vi "Untitled 1.vi"() -> ()   [LabVIEW 2014]
uses:
  <vilib>/addons/control/pid/NI_PID_pid.lvlib
  <vilib>/addons/control/pid/pid.llb/PID (DBL).vi
panel:
  out "Inches Desired 2":dbl
  in  "stop":bool
  out "In Range? 2":bool
  out "Interpolation Error 2":dbl format="%0.2f"
  out "Seconds for Traversal 2":dbl format="%0.2f"
  in  "Inches Desired":dbl(slide) scale=0.0..100.0
  out "Time Required (sec)":dbl
  in  "Distance to Travel (m)":dbl
  out "In Range?":bool
  out "Interpolation Error":dbl format="%0.2f"
  out "Seconds for Traversal":dbl format="%0.2f"
  in  "Watts Available":dbl=1000.0 format="%0.2f"
  in  "PID gains":T1={"proportional gain (Kc)"=1.0, "integral time (Ti, min)"=0.01, "derivative time (Td, min)"=0.0}
  in  "output range":cluster{"output high":dbl, "output low":dbl}={"output high"=1.0, "output low"=0.0}
  in  "process variable":dbl format="%.2f"
  in  "setpoint":dbl format="%.2f"
  out "output to motor":dbl format="%.2f"
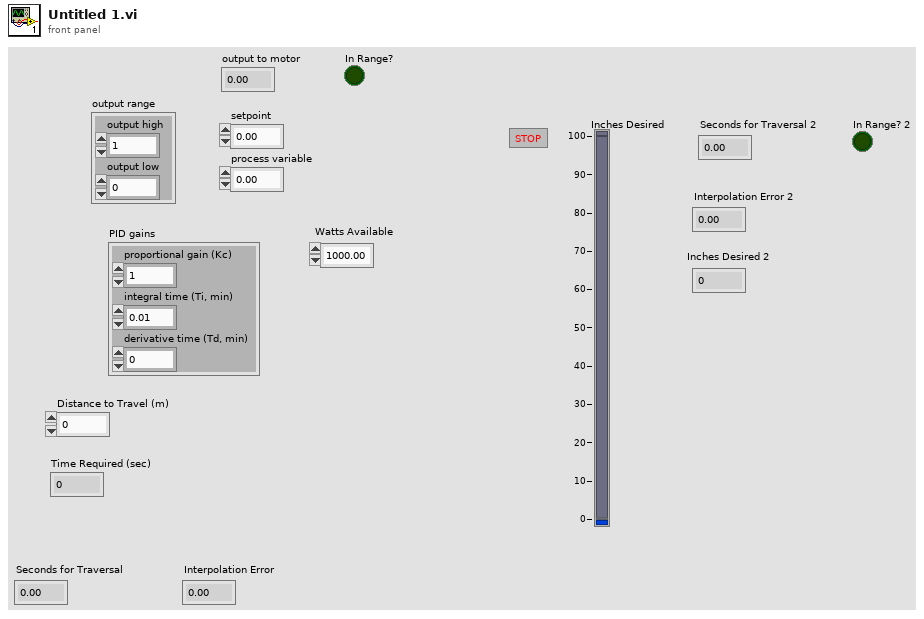
[diagram p1: front panel]
types:
  T1 = cluster{"proportional gain (Kc)":dbl, "integral time (Ti, min)":dbl, "derivative time (Td, min)":dbl}
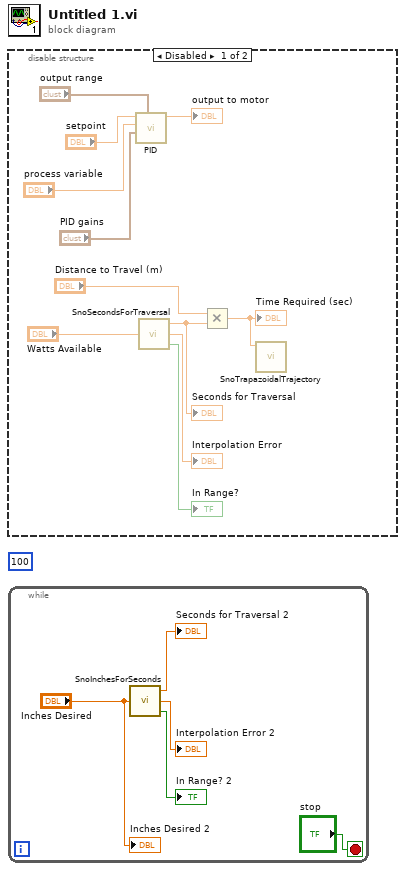
[diagram p0: block diagram]
diagram:
  (unwired) 100
  n1 = disable-structure shown="Disabled" {
    frame Disabled {
      n2 = call-poly <vilib>:"PID.vi"("output range"="output range", "PID gains"="PID gains", "process variable"="process variable", "setpoint"="setpoint") -> ("output"=→"output to motor":dbl)  [unwired: 6 in, 1 out]
      n3 = call "SnoSecondsForTraversal.vi"("Volts Available"="Watts Available") -> ("Seconds for Traversal"=w3:dbl, "Interpolation Error"=→"Interpolation Error":dbl, "In Range?"=→"In Range?":bool)
      "Seconds for Traversal" <- w3
      n4 = Multiply(x="Distance to Travel (m)", y=w3) -> (x*y=w1:dbl)
      "Time Required (sec)" <- w1
      n5 = call "SnoTrapazoidalTrajectory.vi"("Seconds for Traversal"=w1) -> ()  [unwired: 6 in, 1 out]
    }
    frame Enabled {
    }
  }
  n6 = while {
    stop <- "stop" stop-if-true
    n7 = call "SnoInchesForSeconds.vi"("Inches Desired"="Inches Desired") -> ("Seconds for Traversal"=→"Seconds for Traversal 2":dbl, "Interpolation Error"=→"Interpolation Error 2":dbl, "In Range?"=→"In Range? 2":bool)
    "Inches Desired 2" <- "Inches Desired"
  }
